vi "NI32LV223f0ASD1_SAMPLE VI.vi"() -> ()   [LabVIEW 2022 SP3]
panel:
  out "Numeric 3":dbl
  out "Numeric 2":dbl
  out "Numeric":dbl
  in  "?":dbl
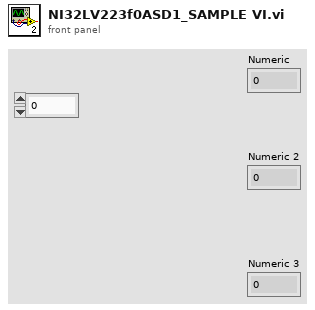
[diagram p1: front panel]
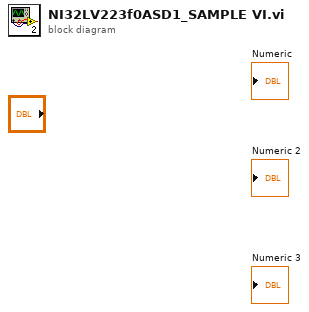
[diagram p0: block diagram]
diagram:
